vi "Clear Error (single).vi"(7 "Convert to Warning (F)":bool, 8 "error in":errorcluster, 11 "Error to Clear":i32) -> (0 "error out":errorcluster, 3 "Cleared Error?":bool)   [LabVIEW 2013]
doc: "Converts up to 4 errors into warnings by passing the error code and text of the error received but setting Status of the error to False. This allows the error information to pass without the VI treating the information as an error."
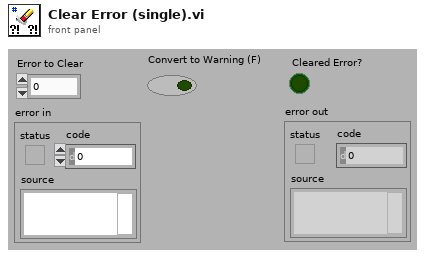
[diagram p1: front panel]
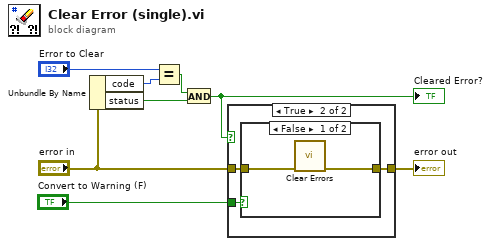
[diagram p0: block diagram]
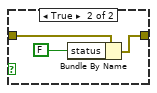
[diagram p3: hidden frame]
diagram:
  n1 = Unbundle By Name("error in") -> ("code"=w2:i32, "status"=w3:bool)
  n2 = Equal?(x="Error to Clear", y=w2) -> (x = y?=w5:bool)
  n3 = And(x=w5, y=w3) -> (x .and. y?=w4:bool)
  "Cleared Error?" <- w4
  n4 = case shown="True" w4 {
    tunnel: "error in" -> [w9 w12]
    tunnel: [w9 w11] -> w7
    tunnel: "Convert to Warning (F)" -> [_ w10]
    frame False {
    }
    frame True {
      n5 = case shown="False" w10 {
        tunnel: w12 -> [w14 w17]
        tunnel: [w13 w16] -> w11
        frame False {
          n6 = call <vilib>:"Clear Errors.vi"("error in (no error)"=w14) -> ("error out"=w13:errorcluster)  [unwired: 6 out]
        }
        frame True {
          n7 = Bundle By Name(cluster=w17, "status"=FALSE) -> (w16:errorcluster)
        }
      }
    }
  }
  "error out" <- w7
